vi "controllockin.vi"(4 "usar multimetro":bool, 6 "Enum":T1(ring), 7 "num lecturas lockin":i32, 8 "Readout Config":string(combo)="POW", 9 "average rate":i32, 10 "tiempo lecturas potenciomtro":i32, 11 "tiempo lecturas lockin":i32) -> (0 "multimetro":dbl format="%0.2f", 1 "valor potenciometro":dbl format="%^#_9e", 2 "Valor Lockin":dbl)   [LabVIEW 2016]
doc: "Este subVI sirve para adquirir la información del lockin y la que se lee desde el potenciómetro en caso de que el ususario la desee.\n\nComo entradas a este subVI son los tiempo de lectura y el número de mediciones del potenciómetro y del lockin. además del tipo de medición que se desea realizar.\n\nComo salida se obtiene el valor que se obtiene del lockin y del potenciómetro."
uses:
  <vilib>/Analysis/baseanly.llb/Mean (DBL).vi
  <vilib>/Analysis/NI_AALBase.lvlib
panel:
  in  "P-DMM":string="16"
  in  "P-LockIn":string="3"
  out "New 2":bool
  out "Error log 2":string
  out "Readout string":string
  out "New":bool
  out "Error log":string
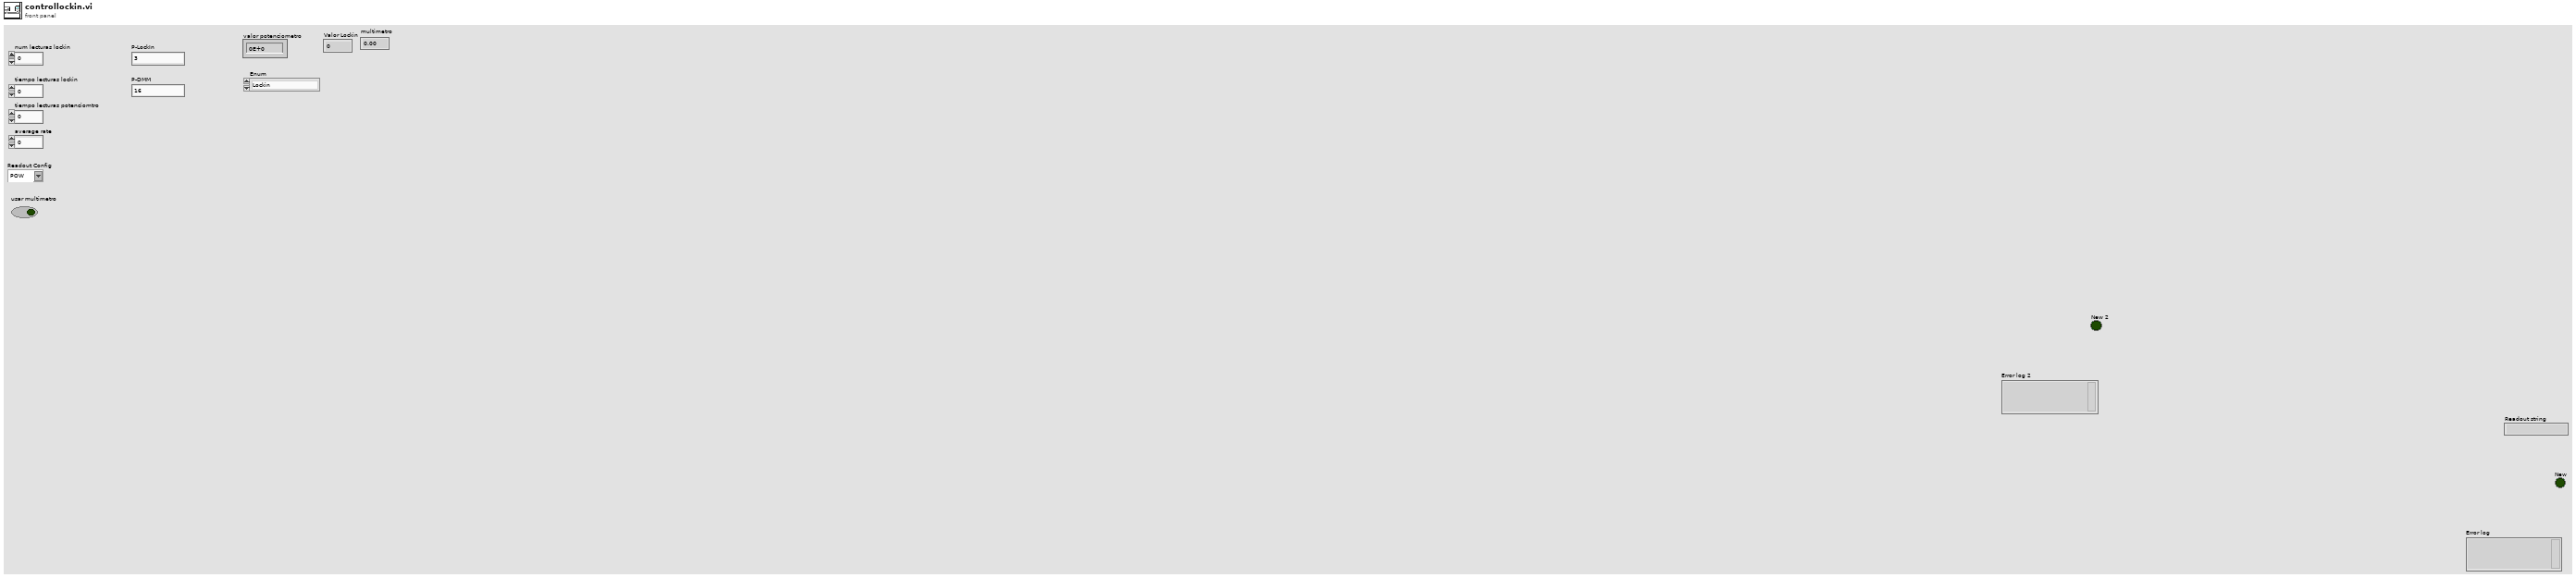
[diagram p1: front panel]
types:
  T1 = enum16{"Lockin", "Lockin-potenciometro", "Potenciometro"}
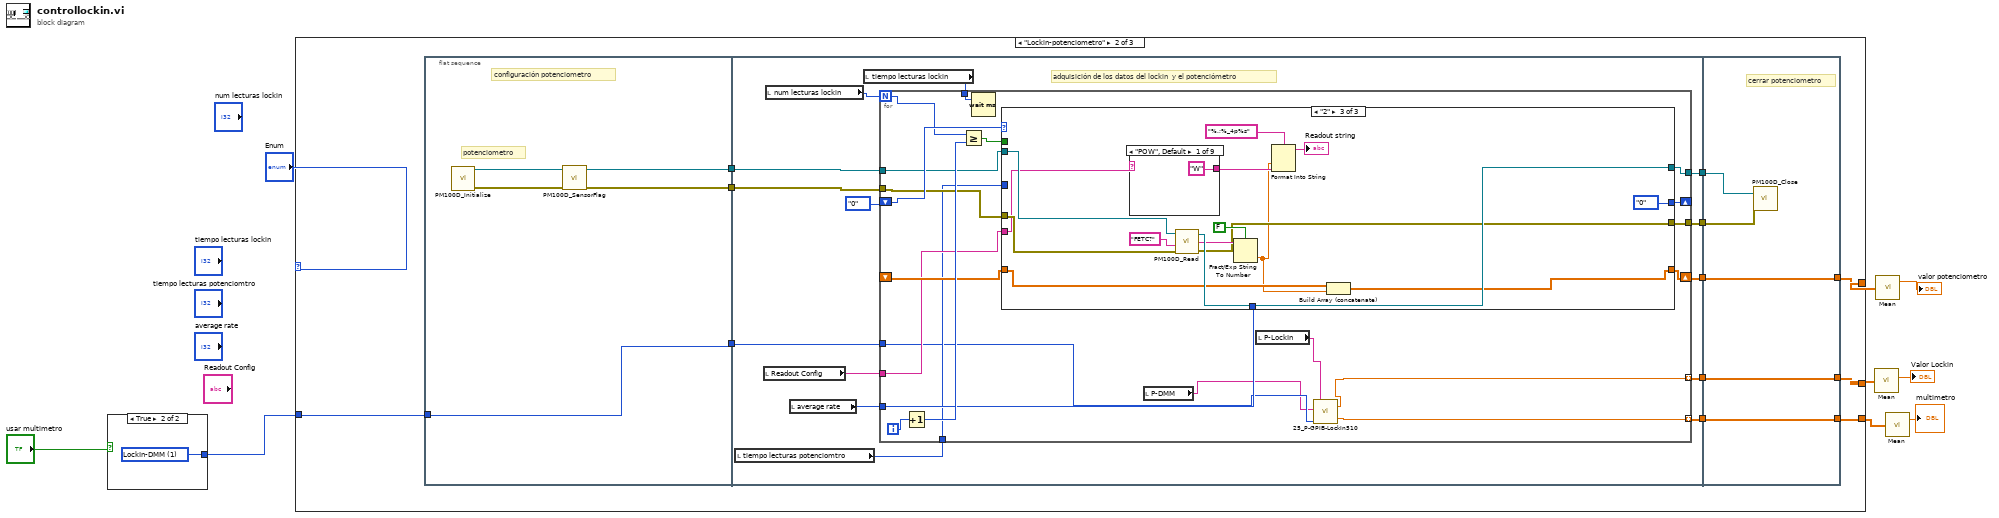
[diagram p0: block diagram]
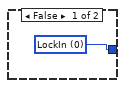
[diagram p2: hidden frame]
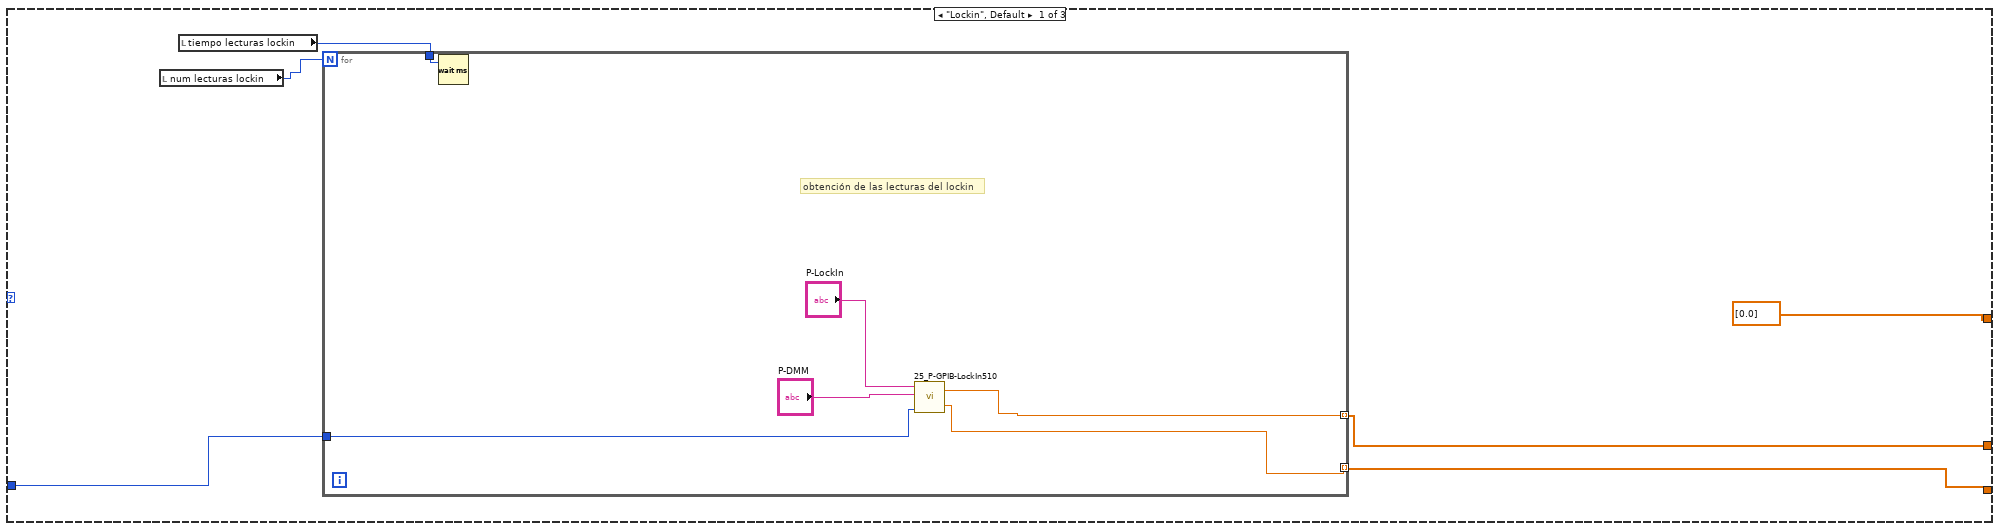
[diagram p3: hidden frame]
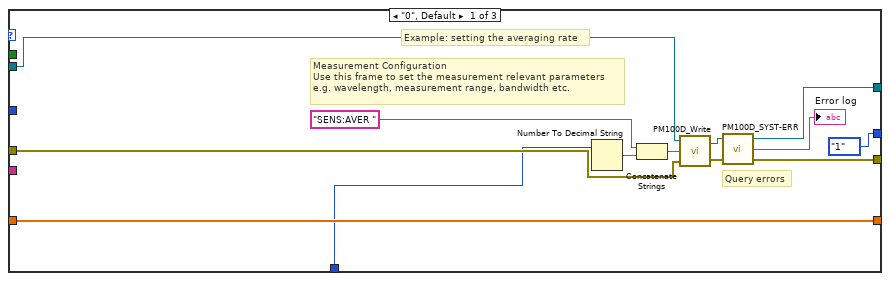
[diagram p4: hidden frame]
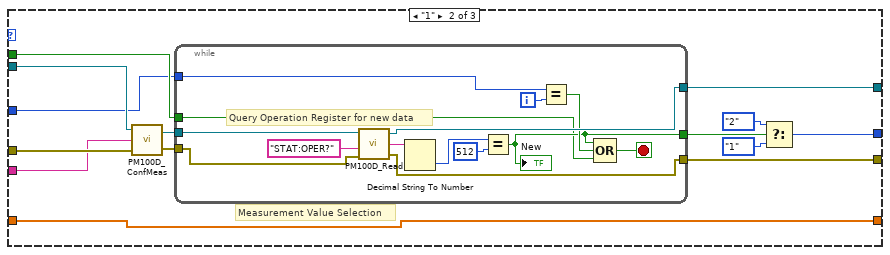
[diagram p5: hidden frame]
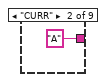
[diagram p6: hidden frame]
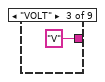
[diagram p7: hidden frame]
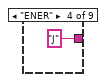
[diagram p8: hidden frame]
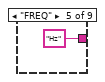
[diagram p9: hidden frame]
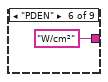
[diagram p10: hidden frame]
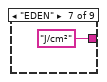
[diagram p11: hidden frame]
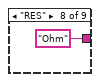
[diagram p12: hidden frame]
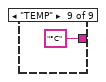
[diagram p13: hidden frame]
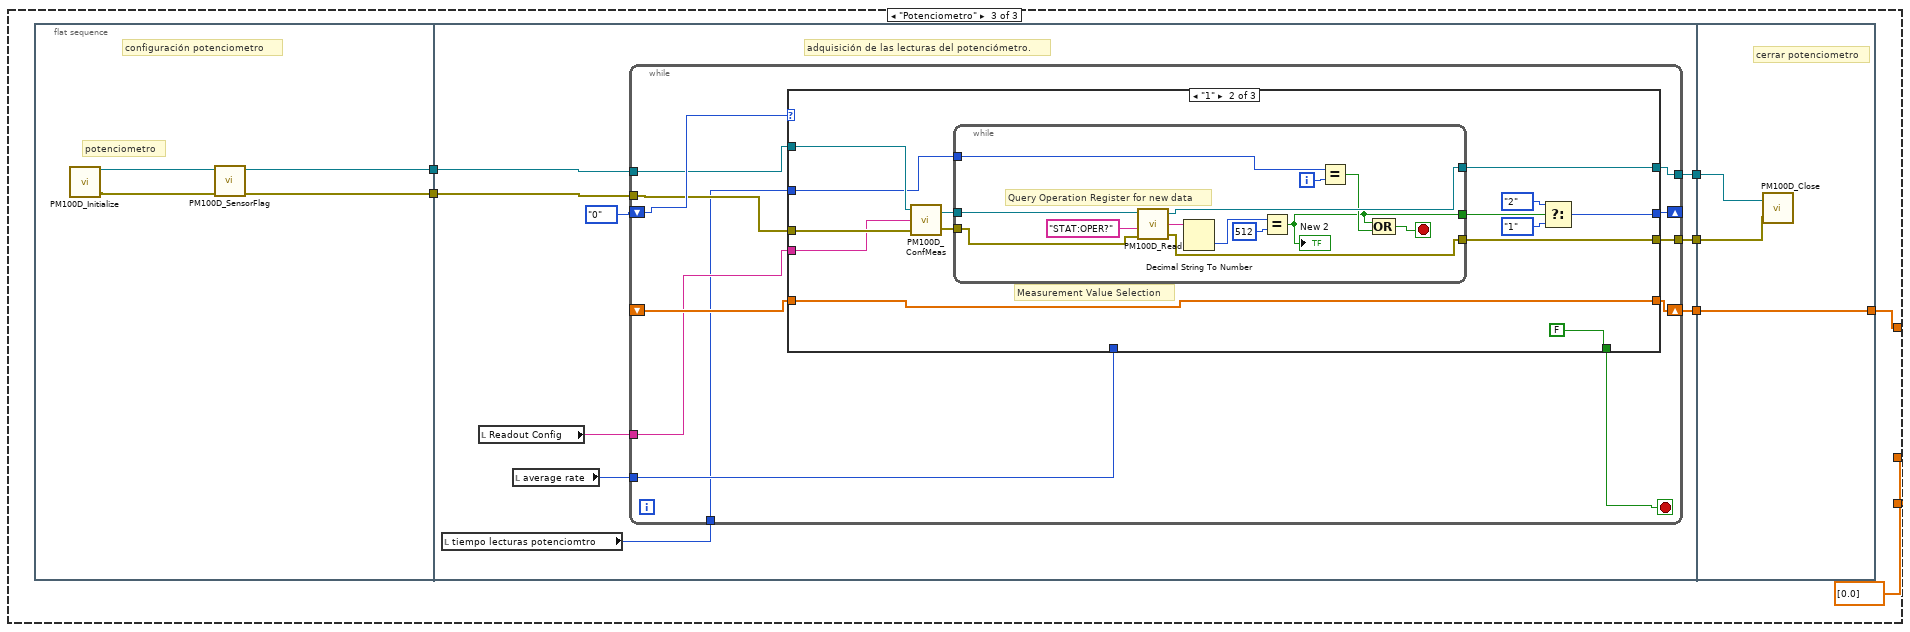
[diagram p14: hidden frame]
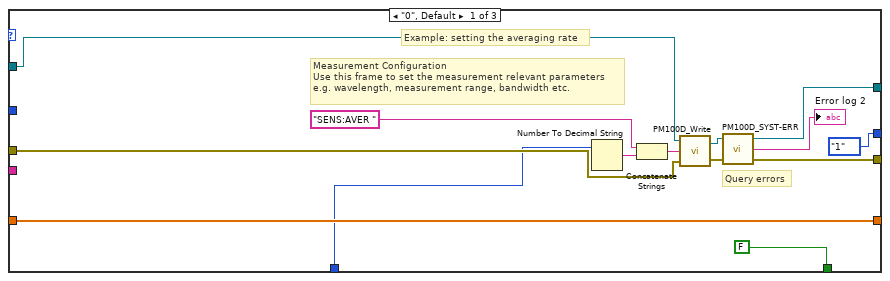
[diagram p15: hidden frame]
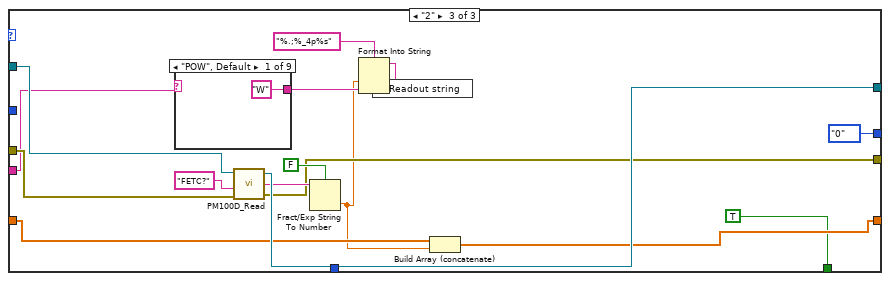
[diagram p16: hidden frame]
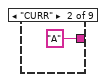
[diagram p17: hidden frame]
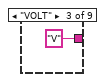
[diagram p18: hidden frame]
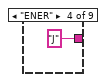
[diagram p19: hidden frame]
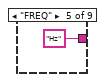
[diagram p20: hidden frame]
diagram:
  n1 = case shown="True" "usar multimetro" {
    tunnel: [w10 w11] -> w4
    frame False {
      w10 = u16 0 items=["LockIn", "LockIn-DMM"] ("Tipo")
    }
    frame True {
      w11 = u16 1 items=["LockIn", "LockIn-DMM"] ("Tipo")
    }
  }
  n2 = case shown="\"Lockin-potenciometro\"" "Enum" {
    tunnel: [dbl[] [0.0] w33 w147] -> w8
    tunnel: [w15 w32 w146] -> w7
    tunnel: w4 -> [w13 w26 _]
    tunnel: [w12 w24 w146] -> w2
    frame "Lockin", Default {
      n3 = local read "num lecturas lockin"() -> (w17:i32)
      n4 = local read "tiempo lecturas lockin"() -> (w16:i32)
      n5 = for {
        N: w17 -> [_]
        tunnel: w16 -> [w23]
        tunnel: [w22] -> w15 mode=indexing
        tunnel: w13 -> [w18]
        tunnel: [w21] -> w12 mode=indexing
        # "obtención de las lecturas del lockin"
        n6 = Wait (ms)(milliseconds to wait=w23) -> ()  [unwired: 1 out]
        n7 = call "25_P-GPIB-LockIn510.vi"("Tipo"=w18, "P-DMM"="P-DMM", "P-LockIn"="P-LockIn") -> ("DMM"=w21:dbl, "LockIn"=w22:dbl)  [unwired: 1 in]
      }
    }
    frame "Lockin-potenciometro" {
      n8 = flat-sequence {
        tunnel: [w38] -> w35
        tunnel: [w37] -> w34
        tunnel: [w36] -> w27
        tunnel: w26 -> [w36]
        tunnel: w35 -> [w54]
        tunnel: w34 -> [w53]
        tunnel: [w46] -> w31
        tunnel: [w45] -> w30
        tunnel: [w44] -> w29
        tunnel: [w43] -> w28
        tunnel: w27 -> [w42]
        tunnel: [w41] -> w25
        tunnel: [w144] -> w32
        tunnel: [w145] -> w33
        tunnel: w31 -> [w145]
        tunnel: w30 -> [w144]
        tunnel: w29 -> [w143]
        tunnel: w28 -> [w142]
        tunnel: w25 -> [w141]
        tunnel: [w141] -> w24
        frame #0 {
          # "potenciometro"
          # "configuración potenciometro"
          n9 = call "PM100D_Initialize.vi"() -> ("error out"=w40:errorcluster, "VISA out"=w39:refnum<visa-resource-name>)  [unwired: 2 in, 2 out]
          n10 = call "PM100D_SensorFlag.vi"("error in (no error)"=w40, "VISA in"=w39) -> ("error out"=w37:errorcluster, "VISA out"=w38:refnum<visa-resource-name>)  [unwired: 2 in, 6 out]
        }
        frame #1 {
          # "adquisición de los datos del lockin  y el potenciómetro"
          n11 = local read "tiempo lecturas potenciomtro"() -> (w47:i32)
          n12 = local read "Readout Config"() -> (w49:string)
          n13 = local read "num lecturas lockin"() -> (w52:i32)
          n14 = local read "average rate"() -> (w48:i32)
          n15 = local read "tiempo lecturas lockin"() -> (w51:i32)
          n16 = for {
            N: w52 -> [w72]
            tunnel: w54 -> [w69]
            tunnel: w53 -> [w68]
            tunnel: w51 -> [w75]
            shift-right: [w62] -> _
            shift-left: enum16{"0", "1", "2"}."0" ("f") -> [w74]
            shift-right: [w66] -> w46
            shift-left: _ -> [w67]
            tunnel: w49 -> [w65]
            tunnel: w48 -> [w64]
            tunnel: w47 -> [w63]
            tunnel: [w56] -> w45 mode=indexing
            tunnel: [w61] -> w44
            tunnel: [w60] -> w43
            tunnel: w42 -> [w59]
            tunnel: [w55] -> w41 mode=indexing
            i -> [w71]
            n17 = Increment(x=w71) -> (x+1=w70:i32)
            n18 = Greater Or Equal?(x=w72, y=w70) -> (x >= y?=w73:bool)
            n19 = Wait (ms)(milliseconds to wait=w75) -> ()  [unwired: 1 out]
            n20 = case shown="\"2\"" w74 {
              tunnel: w69 -> [w86 w102 w129]
              tunnel: w68 -> [w81 w101 w128]
              tunnel: [enum16{"0", "1", "2"}."1" w96 enum16{"0", "1", "2"}."0"] -> w62
              tunnel: [w79 w98 w127] -> w61
              tunnel: [w78 w97 w122] -> w60
              tunnel: w73 -> [_ w92 _]
              tunnel: w67 -> [w77 w91 w121]
              tunnel: [w77 w91 w119] -> w66
              tunnel: w65 -> [_ w90 w118]
              tunnel: w63 -> [_ w89 _]
              tunnel: w64 -> [w76 _ _]
              frame "0", Default {
                # "Query errors"
                # "Example: setting the averaging rate"
                # "Measurement Configuration\nUse this frame to set the measurement relevant parameters\ne.g. wavelength, measurement range, bandwidth etc."
                n21 = Number To Decimal String(number=w76) -> (decimal integer string=w87:string)  [unwired: 1 in]
                n22 = Concatenate Strings("SENS:AVER " ("string"), w87) -> (w85:string)
                n23 = call "PM100D_Write.vi"("error in (no error)"=w81, "Command"=w85, "VISA in"=w86) -> ("error out"=w82:errorcluster, "VISA out"=w84:refnum<visa-resource-name>)
                n24 = call "PM100D_SYST-ERR.vi"("error out 2"=w82, "VISA In"=w84) -> ("error out"=w78:errorcluster, "Error"=→"Error log":string, "VISA Out"=w79:refnum<visa-resource-name>)  [unwired: 1 in]
              }
              frame "1" {
                # "Measurement Value Selection"
                n25 = call "PM100D_ConfMeas.vi"("error in"=w101, "Conf:"=w90, "VISA In"=w102) -> ("error out"=w99:errorcluster, "dup VISA session"=w100:refnum<visa-resource-name>)
                n26 = while {
                  tunnel: w100 -> [w112]
                  tunnel: w99 -> [w111]
                  tunnel: [w110] -> w98
                  tunnel: [w109] -> w97
                  tunnel: [w105] -> w93
                  tunnel: w92 -> [w104]
                  tunnel: w89 -> [w103]
                  i -> [w107]
                  stop <- w108 stop-if-true
                  # "Query Operation Register for new data"
                  n27 = call "PM100D_Read.vi"("error in (no error)"=w111, "Command"="STAT:OPER?", "VISA in"=w112) -> ("error out"=w109:errorcluster, "ReadValue"=w115:string, "VISA out"=w110:refnum<visa-resource-name>)  [unwired: 1 in]
                  n28 = Decimal String To Number(string=w115) -> (number=w114:i32)  [unwired: 2 in, 1 out]
                  n29 = Equal?(x=w114, y=512) -> (x = y?=w105:bool)
                  "New" <- w105
                  n30 = Equal?(x=w103, y=w107) -> (x = y?=w106:bool)
                  n31 = Compound Arithmetic op=OR(w105, w106, w104) -> (w108:bool)
                }
                n32 = Select(t=enum16{"0", "1", "2"}."2", s=w93, f=enum16{"0", "1", "2"}."1") -> (s? t:f=w96:enum16{"0", "1", "2"})
              }
              frame "2" {
                n33 = case shown="\"POW\", Default" w118 {
                  tunnel: ["W" "A" "V" "J" "Hz" "W/cm²" "J/cm²" "Ohm" "°C"] -> w124
                  frame "POW", Default {
                  }
                  frame "CURR" {
                  }
                  frame "VOLT" {
                  }
                  frame "ENER" {
                  }
                  frame "FREQ" {
                  }
                  frame "PDEN" {
                  }
                  frame "EDEN" {
                  }
                  frame "RES" {
                  }
                  frame "TEMP" {
                  }
                }
                n34 = call "PM100D_Read.vi"("error in (no error)"=w128, "Command"="FETC?", "VISA in"=w129) -> ("error out"=w122:errorcluster, "ReadValue"=w126:string, "VISA out"=w127:refnum<visa-resource-name>)  [unwired: 1 in]
                n35 = Fract/Exp String To Number(use system decimal point (T)=FALSE, string=w126) -> (number=w120:dbl)  [unwired: 2 in, 1 out]
                n36 = Format Into String(format string="%.;%_4p%s", w120, w124) -> (resulting string=→"Readout string":string)  [unwired: 2 in, 1 out]
                n37 = Build Array (concatenate)(w121, w120) -> (w119:dbl[])
              }
            }
            n38 = local read "P-DMM"() -> (w57:string)
            n39 = local read "P-LockIn"() -> (w58:string)
            n40 = call "25_P-GPIB-LockIn510.vi"("Tipo"=w59, "P-DMM"=w57, "P-LockIn"=w58) -> ("DMM"=w55:dbl, "LockIn"=w56:dbl)  [unwired: 1 in]
          }
        }
        frame #2 {
          # "cerrar potenciometro"
          n41 = call "PM100D_Close.vi"("error in (no error)"=w142, "VISA resource name"=w143) -> ()  [unwired: 2 in]
        }
      }
    }
    frame "Potenciometro" {
      w146 = dbl[] [0.0]
      n42 = flat-sequence {
        tunnel: [w154] -> w152
        tunnel: [w153] -> w151
        tunnel: w152 -> [w165]
        tunnel: w151 -> [w164]
        tunnel: [w159] -> w150
        tunnel: [w158] -> w149
        tunnel: [w157] -> w148
        tunnel: [w246] -> w147
        tunnel: w150 -> [w246]
        tunnel: w149 -> [w245]
        tunnel: w148 -> [w244]
        frame #0 {
          # "potenciometro"
          # "configuración potenciometro"
          n43 = call "PM100D_Initialize.vi"() -> ("error out"=w156:errorcluster, "VISA out"=w155:refnum<visa-resource-name>)  [unwired: 2 in, 2 out]
          n44 = call "PM100D_SensorFlag.vi"("error in (no error)"=w156, "VISA in"=w155) -> ("error out"=w153:errorcluster, "VISA out"=w154:refnum<visa-resource-name>)  [unwired: 2 in, 6 out]
        }
        frame #1 {
          # "adquisición de las lecturas del potenciómetro."
          n45 = local read "tiempo lecturas potenciomtro"() -> (w160:i32)
          n46 = local read "Readout Config"() -> (w162:string)
          n47 = local read "average rate"() -> (w161:i32)
          n48 = while {
            tunnel: w165 -> [w176]
            tunnel: w164 -> [w175]
            shift-right: [w169] -> _
            shift-left: enum16{"0", "1", "2"}."0" ("f") -> [w177]
            shift-right: [w173] -> w159
            shift-left: _ -> [w174]
            tunnel: w162 -> [w172]
            tunnel: w161 -> [w171]
            tunnel: w160 -> [w170]
            tunnel: [w168] -> w158
            tunnel: [w167] -> w157
            stop <- w166 stop-if-true
            n49 = case shown="\"1\"" w177 {
              tunnel: w176 -> [w189 w205 w232]
              tunnel: w175 -> [w184 w204 w231]
              tunnel: [enum16{"0", "1", "2"}."1" w199 enum16{"0", "1", "2"}."0"] -> w169
              tunnel: [w182 w201 w230] -> w168
              tunnel: [w181 w200 w225] -> w167
              tunnel: w174 -> [w180 w195 w224]
              tunnel: [w180 w195 w222] -> w173
              tunnel: w172 -> [_ w194 w221]
              tunnel: w170 -> [_ w193 _]
              tunnel: w171 -> [w179 _ _]
              tunnel: [FALSE FALSE TRUE] -> w166
              frame "0", Default {
                # "Query errors"
                # "Example: setting the averaging rate"
                # "Measurement Configuration\nUse this frame to set the measurement relevant parameters\ne.g. wavelength, measurement range, bandwidth etc."
                n50 = Number To Decimal String(number=w179) -> (decimal integer string=w190:string)  [unwired: 1 in]
                n51 = Concatenate Strings("SENS:AVER " ("string"), w190) -> (w188:string)
                n52 = call "PM100D_Write.vi"("error in (no error)"=w184, "Command"=w188, "VISA in"=w189) -> ("error out"=w185:errorcluster, "VISA out"=w187:refnum<visa-resource-name>)
                n53 = call "PM100D_SYST-ERR.vi"("error out 2"=w185, "VISA In"=w187) -> ("error out"=w181:errorcluster, "Error"=→"Error log 2":string, "VISA Out"=w182:refnum<visa-resource-name>)  [unwired: 1 in]
              }
              frame "1" {
                # "Measurement Value Selection"
                n54 = call "PM100D_ConfMeas.vi"("error in"=w204, "Conf:"=w194, "VISA In"=w205) -> ("error out"=w202:errorcluster, "dup VISA session"=w203:refnum<visa-resource-name>)
                n55 = while {
                  tunnel: w203 -> [w214]
                  tunnel: w202 -> [w213]
                  tunnel: [w212] -> w201
                  tunnel: [w211] -> w200
                  tunnel: [w207] -> w196
                  tunnel: w193 -> [w206]
                  i -> [w209]
                  stop <- w210 stop-if-true
                  # "Query Operation Register for new data"
                  n56 = call "PM100D_Read.vi"("error in (no error)"=w213, "Command"="STAT:OPER?", "VISA in"=w214) -> ("error out"=w211:errorcluster, "ReadValue"=w217:string, "VISA out"=w212:refnum<visa-resource-name>)  [unwired: 1 in]
                  n57 = Decimal String To Number(string=w217) -> (number=w216:i32)  [unwired: 2 in, 1 out]
                  n58 = Equal?(x=w216, y=512) -> (x = y?=w207:bool)
                  "New 2" <- w207
                  n59 = Equal?(x=w206, y=w209) -> (x = y?=w208:bool)
                  n60 = Compound Arithmetic op=OR(w207, w208) -> (w210:bool)
                }
                n61 = Select(t=enum16{"0", "1", "2"}."2", s=w196, f=enum16{"0", "1", "2"}."1") -> (s? t:f=w199:enum16{"0", "1", "2"})
              }
              frame "2" {
                n62 = case shown="\"POW\", Default" w221 {
                  tunnel: ["W" "A" "V" "J" "Hz" "W/cm²" "J/cm²" "Ohm" "°C"] -> w227
                  frame "POW", Default {
                  }
                  frame "CURR" {
                  }
                  frame "VOLT" {
                  }
                  frame "ENER" {
                  }
                  frame "FREQ" {
                  }
                  frame "PDEN" {
                  }
                  frame "EDEN" {
                  }
                  frame "RES" {
                  }
                  frame "TEMP" {
                  }
                }
                n63 = call "PM100D_Read.vi"("error in (no error)"=w231, "Command"="FETC?", "VISA in"=w232) -> ("error out"=w225:errorcluster, "ReadValue"=w229:string, "VISA out"=w230:refnum<visa-resource-name>)  [unwired: 1 in]
                n64 = Fract/Exp String To Number(use system decimal point (T)=FALSE, string=w229) -> (number=w223:dbl)  [unwired: 2 in, 1 out]
                n65 = Format Into String(format string="%.;%_4p%s", w223, w227) -> (resulting string=w220:string)  [unwired: 2 in, 1 out]
                n66 = local write "Readout string"(w220) -> ()
                n67 = Build Array (concatenate)(w224, w223) -> (w222:dbl[])
              }
            }
          }
        }
        frame #2 {
          # "cerrar potenciometro"
          n68 = call "PM100D_Close.vi"("error in (no error)"=w244, "VISA resource name"=w245) -> ()  [unwired: 2 in]
        }
      }
    }
  }
  n69 = call-poly <vilib>:"Mean.vi"("X"=w7) -> ("mean"=→"Valor Lockin":dbl)  [unwired: 1 out]
  n70 = call-poly <vilib>:"Mean.vi"("X"=w8) -> ("mean"=→"valor potenciometro":dbl)  [unwired: 1 out]
  n71 = call-poly <vilib>:"Mean.vi"("X"=w2) -> ("mean"=→"multimetro":dbl)  [unwired: 1 out]
